vi "GET_security_access_status.vi"() -> ()   [LabVIEW 2024]
uses:
  <vilib>/httpClient/LabVIEWHTTPClient.lvlib
panel:
  out "value":T1
  in  "API Key":string="cheia04042025tema2restfulapi"
  out "headers":string
  out "error out json":errorcluster
  out "body":string
  out "error out get":errorcluster
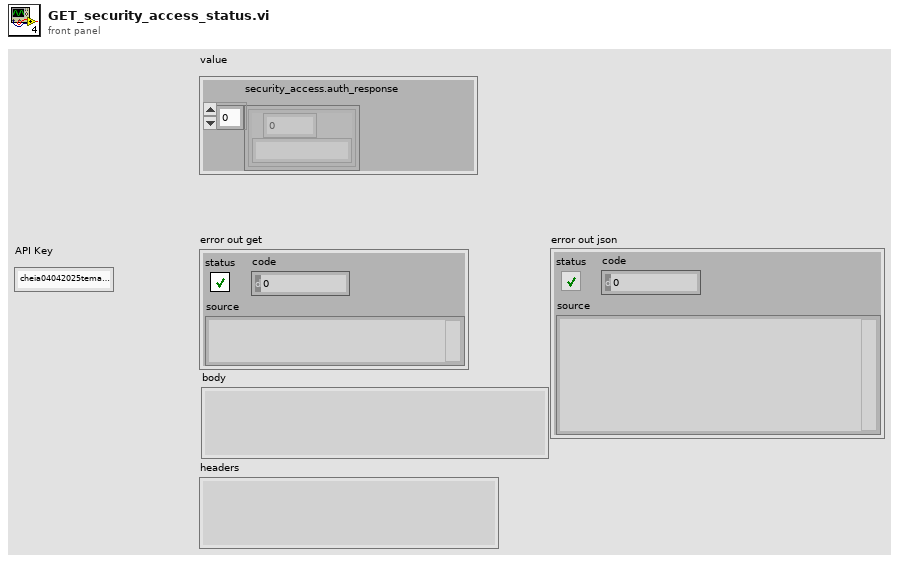
[diagram p1: front panel]
types:
  T1 = cluster{"security_access.auth_response":cluster{dbl, string}[]}
  T2 = typedef "LabVIEWHTTPClient.lvlib/ClientHandle.ctl" = refnum<k1>
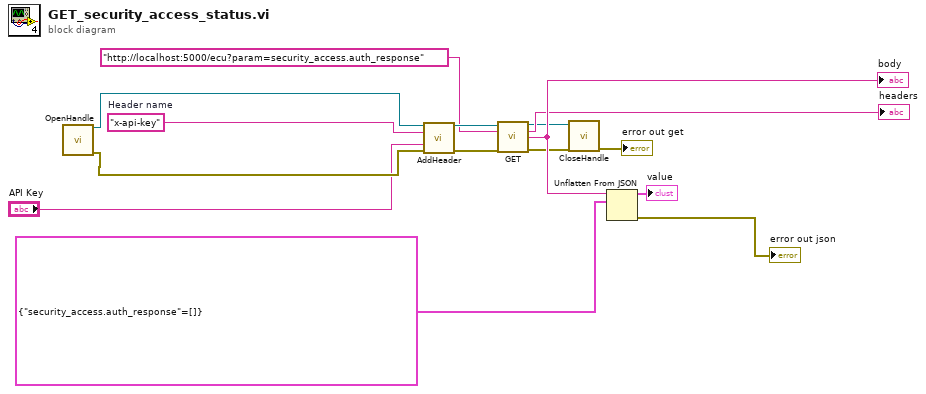
[diagram p0: block diagram]
diagram:
  w5 = "x-api-key"  # Header name
  n1 = call <vilib>:"OpenHandle.vi"() -> ("client handle out"=w6:T2, "error out"=w7:errorcluster)  [unwired: 14 in]
  n2 = call <vilib>:"AddHeader.vi"("client handle"=w6, "header"=w5, "value"="API Key", "error in (no error)"=w7) -> ("client handle out"=w9:T2, "error out"=w8:errorcluster)  [unwired: 10 in]
  n3 = call <vilib>:"GET.vi"("client handle"=w9, "url"="http://localhost:5000/ecu?param=security_access.auth_response", "error in (no error)"=w8) -> ("client handle out"=w11:T2, "headers"=→"headers":string, "body"=w15:string, "error out"=w10:errorcluster)  [unwired: 9 in]
  "body" <- w15
  n4 = call <vilib>:"CloseHandle.vi"("client handle"=w11, "error in (no error)"=w10) -> ("error out"=→"error out get":errorcluster)  [unwired: 13 in]
  n5 = Unflatten From JSON(JSON string=w15, type and defaults=T1 {"security_access.auth_response"=[]}) -> (value=→"value":T1, error out=→"error out json":errorcluster)  [unwired: 5 in]
